vi "_emi_Start Loop Array.vi"(2 "Start even on error(T)":bool=TRUE, 5 "Loop IDs in":u16[](array[numeric]), 7 "Allow start(T)":bool=TRUE, 9 "error in (no error)":errorcluster) -> (6 "Loop IDs out":u16[](array[numeric]), 10 "error out":errorcluster, 13 "Start loop":bool)   [LabVIEW 2010]
doc: "Check wheter a loop should start. based on loop enable(Loop control),\n\nExecutes as normal on error"
uses:
  Basic/0 - General/Error/emi_Is Error.vi
  _emi_GFV stop a loop so it can reset.vi
  _emi_GFV Loop Linking.vi
  _emi_GFV Loop Enable.vi
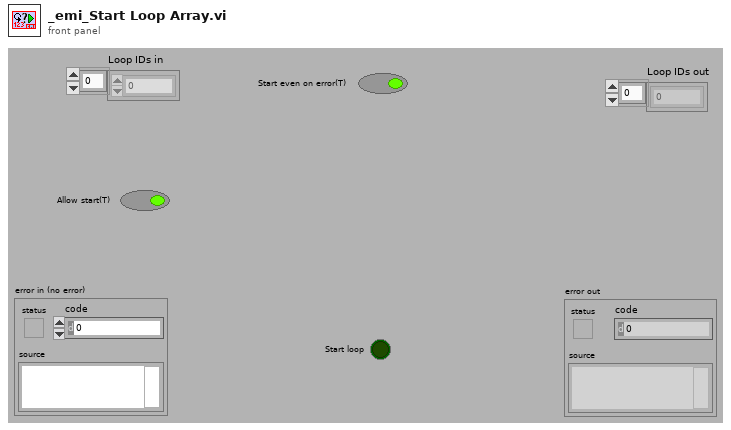
[diagram p1: front panel]
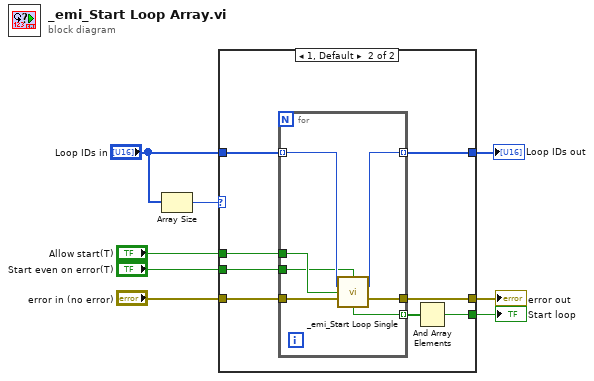
[diagram p0: block diagram]
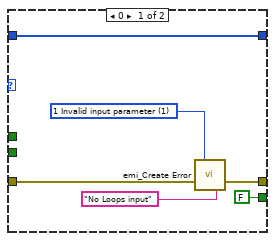
[diagram p2: hidden frame]
diagram:
  n1 = Array Size(array="Loop IDs in") -> (size(s)=w6:i32)
  n2 = case shown="1, Default" w6 {
    tunnel: "error in (no error)" -> [w14 w22]
    tunnel: [w13 w21] -> w7
    tunnel: [w10 w19] -> w5
    tunnel: "Loop IDs in" -> [w10 w20]
    tunnel: "Allow start(T)" -> [_ w18]
    tunnel: "Start even on error(T)" -> [_ w17]
    tunnel: [FALSE w15] -> w1
    frame 0 {
      w12 = 1 items=["0 No Error"=0, "1 Invalid input parameter"=1, "6 Generic file IO "=6, "7 File not Found"=7, "35 Generic Pring Error"=35, "37 Device not Found"=37, "39 Device Unit Error"=39, "40 Could fot Open Device"=40, "42 Generic Error"=42, "52 Unknown Message"=52, "98 Bad File type"=98, "99 Bad File Version"=99, "100 Bad Data in File"=100, "1018 Unspecefied Error"=1018, "1041 Incorrect Password"=1041, "1043 Feature not in this version"=1043, "1109 Unsuported Data type"=1109, "1444 Did not close sucessfully"=1444] ("Error Code")
      n3 = call "emi_Create Error.vi"("Error Code"=w12, "error in (no error)"=w14, "Append String(\"\")"="No Loops input" ("Append String(\"\")")) -> ("error out"=w13:errorcluster)  [unwired: 12 in]
    }
    frame 1, Default {
      n4 = for {
        tunnel: w22 -> [w29]
        tunnel: [w28] -> w21
        tunnel: w20 -> [w27] mode=indexing
        tunnel: [w26] -> w19 mode=indexing
        tunnel: w18 -> [w25]
        tunnel: w17 -> [w24]
        tunnel: [w23] -> w16 mode=indexing
        n5 = call "_emi_Start Loop Single.vi"("Start even on error(T)"=w24, "Loop ID in"=w27, "Allow start(T)"=w25, "error in (no error)"=w29) -> ("Loop ID out"=w26:u16, "error out"=w28:errorcluster, "Start loop"=w23:bool)  [unwired: 9 in]
      }
      n6 = And Array Elements(Boolean array=w16) -> (logical AND=w15:bool)
    }
  }
  "error out" <- w7
  "Start loop" <- w1
  "Loop IDs out" <- w5
